vi "BRig_dataCurrent_LaserSwitch_l1.vi"() -> (2 "output_LaserSwitch_l1":i32)   [LabVIEW 2014]
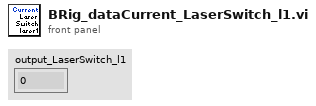
[diagram p1: front panel]
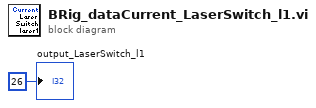
[diagram p0: block diagram]
diagram:
  "output_LaserSwitch_l1" <- 26 ("output_iBlock")
